vi "计算5针真维度.vi"(2 "引用句柄输入":T2, 3 "Fitted Circle (中间圆)":T1, 4 "Fitted Circle (右下角圆)":T1, 5 "Fitted Circle (左下角圆)":T1, 6 "Fitted Circle (右上角圆)":T1, 7 "Fitted Circle (左上角圆)":T1) -> (1 "Distances":sgl[][](array[numeric]))   [LabVIEW 2014]
uses:
  <vilib>/vision/Image Controls.llb/IMAQ Image.ctl
  <vilib>/vision/NI_Vision_Development_Module.lvlib
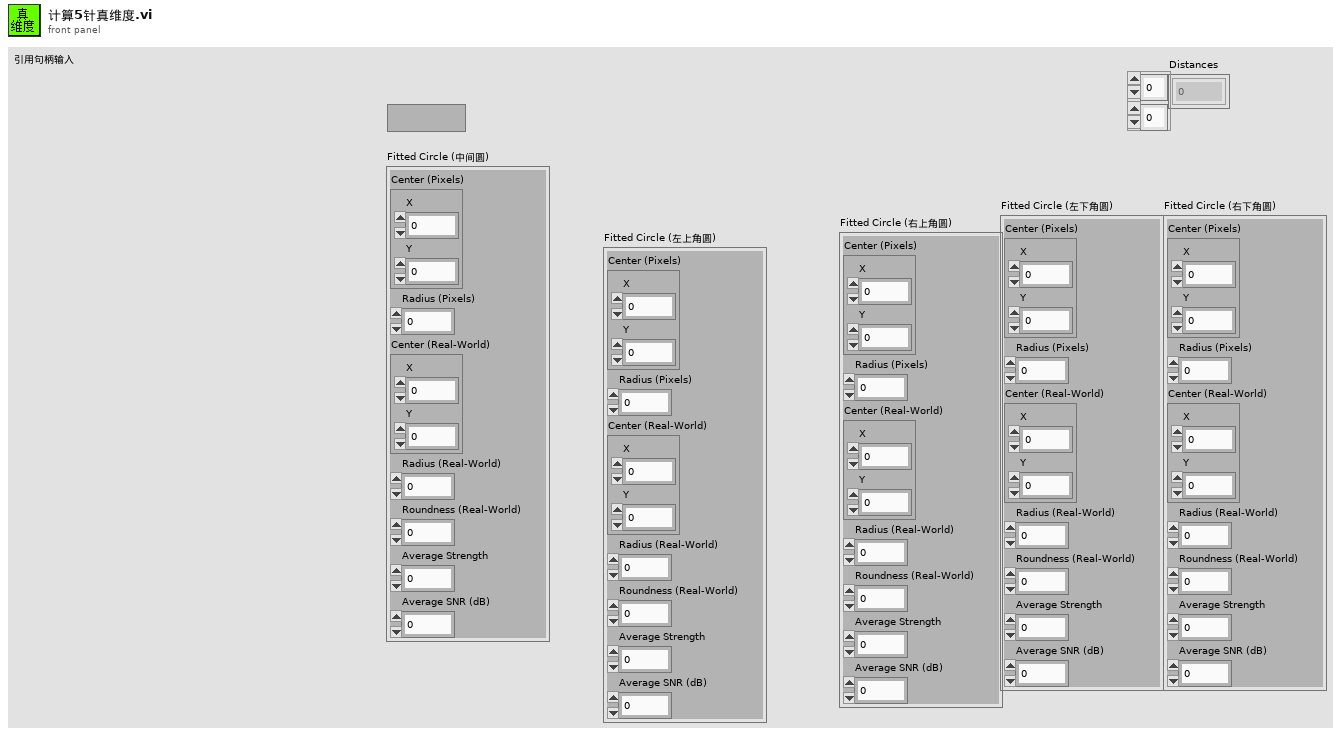
[diagram p1: front panel]
types:
  T1 = cluster{"Center (Pixels)":cluster{"X":sgl, "Y":sgl}, "Radius (Pixels)":dbl, "Center (Real-World)":cluster{"X":sgl, "Y":sgl}, "Radius (Real-World)":dbl, "Roundness (Real-World)":dbl, "Average Strength":dbl, "Average SNR (dB)":dbl}
  T2 = typedef "IMAQ Image.ctl" = refnum<image>
  T3 = cluster{"Center (Pixels)":cluster{"X":sgl, "Y":sgl}, "Radius (Pixels)":dbl, "Center (Real-World)":cluster{"X":sgl, "Y":sgl}, "Radius (Real-World)":dbl, "Roundness (Real-World)":dbl, "Average Strength":dbl, "Average SNR (dB)":dbl}[]
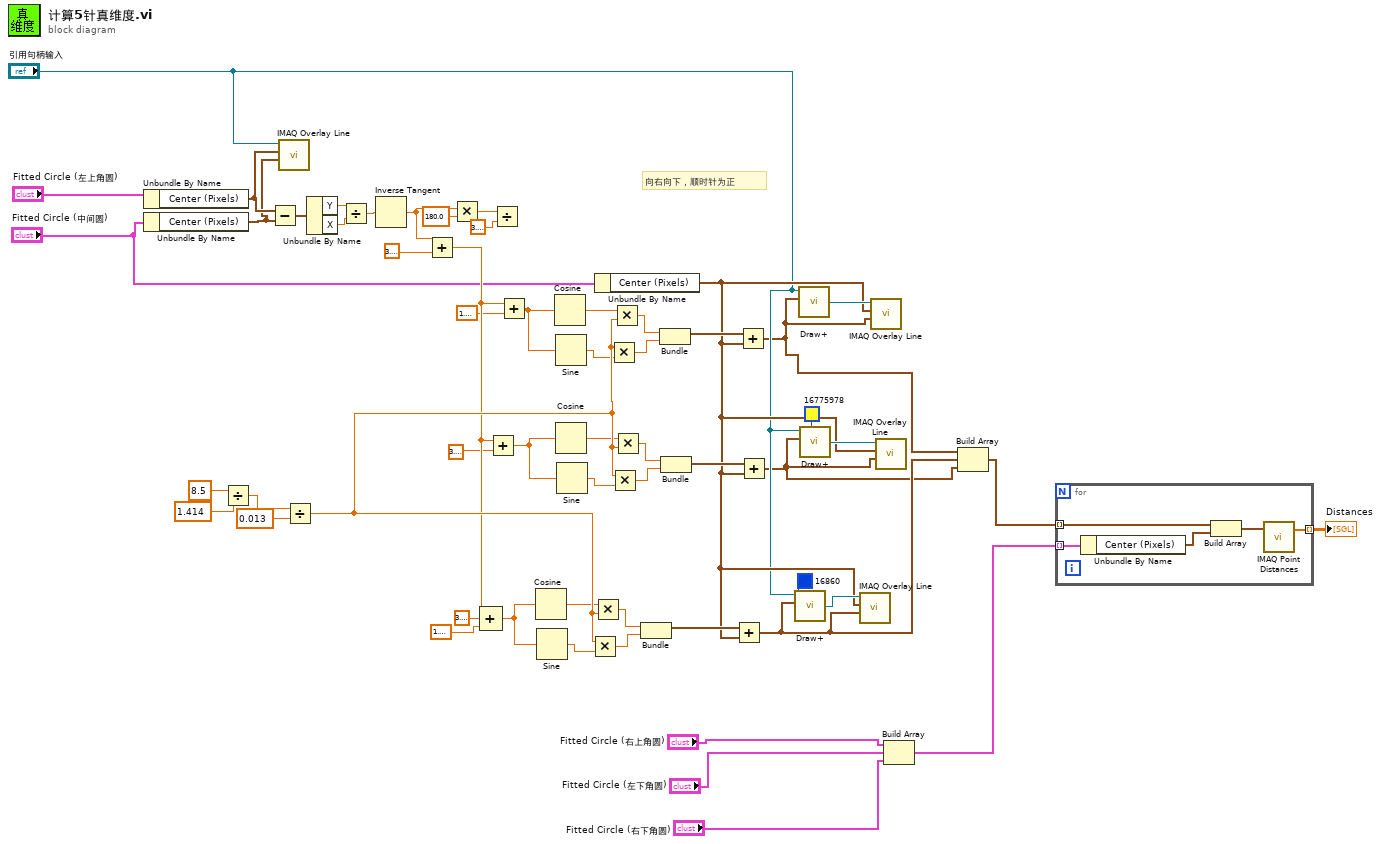
[diagram p0: block diagram]
diagram:
  # "向右向下，顺时针为正"
  n1 = Unbundle By Name("Fitted Circle (左上角圆)") -> ("Center (Pixels)"=w11:cluster{"X":sgl, "Y":sgl})
  n2 = Unbundle By Name("Fitted Circle (中间圆)") -> ("Center (Pixels)"=w10:cluster{"X":sgl, "Y":sgl})
  n3 = Divide(x=8.5, y=1.414) -> (x/y=w26:dbl)
  n4 = Subtract(x=w11, y=w10) -> (x-y=w41:cluster{"X":sgl, "Y":sgl})
  n5 = call "IMAQ Overlay Line"("End Point"=w10, "Start Point"=w11, "Image"="引用句柄输入") -> ()  [unwired: 7 in, 2 out]
  n6 = Divide(x=w26, y=0.013) -> (x/y=w53:dbl)
  n7 = Unbundle By Name(w41) -> ("Y"=w42:sgl, "X"=w43:sgl)
  n8 = Divide(x=w42, y=w43) -> (x/y=w56:sgl)
  n9 = Inverse Tangent(1:w56) -> (0:w57:sgl)
  n10 = Add(x=w57, y=3.141592653589793) -> (x+y=w49:dbl)
  n11 = Multiply(x=w57, y=sgl 180.0) -> (x*y=w19:sgl)
  n12 = Compound Arithmetic op=ADD(w49, 3.141592653589793, 1.5707963267948966) -> (w35:dbl)
  n13 = Add(x=w49, y=3.141592653589793) -> (x+y=w50:dbl)
  n14 = Divide(x=w19, y=3.141592653589793) -> ()  [unwired: 1 out]
  n15 = Add(x=w49, y=1.5707963267948966) -> (x+y=w34:dbl)
  n16 = Cosine(x=w35) -> (cos(x)=w46:dbl)
  n17 = Sine(x=w35) -> (sin(x)=w47:dbl)
  n18 = Cosine(x=w34) -> (cos(x)=w44:dbl)
  n19 = Sine(x=w34) -> (sin(x)=w45:dbl)
  n20 = Cosine(x=w50) -> (cos(x)=w51:dbl)
  n21 = Sine(x=w50) -> (sin(x)=w52:dbl)
  n22 = Multiply(x=w53, y=w47) -> (x*y=w32:dbl)
  n23 = Multiply(x=w46, y=w53) -> (x*y=w31:dbl)
  n24 = Unbundle By Name("Fitted Circle (中间圆)") -> ("Center (Pixels)"=w13:cluster{"X":sgl, "Y":sgl})
  n25 = Multiply(x=w53, y=w45) -> (x*y=w25:dbl)
  n26 = Multiply(x=w53, y=w52) -> (x*y=w54:dbl)
  n27 = Multiply(x=w44, y=w53) -> (x*y=w24:dbl)
  n28 = Multiply(x=w51, y=w53) -> (x*y=w55:dbl)
  n29 = Bundle(w31, w32) -> (w33:cluster{dbl, dbl})  [unwired: 1 in]
  n30 = Bundle(w24, w25) -> (w29:cluster{dbl, dbl})  [unwired: 1 in]
  n31 = Bundle(w55, w54) -> (w30:cluster{dbl, dbl})  [unwired: 1 in]
  n32 = Add(x=w33, y=w13) -> (x+y=w5:cluster{dbl, dbl})
  n33 = Add(x=w29, y=w13) -> (x+y=w6:cluster{dbl, dbl})
  n34 = Add(x=w30, y=w13) -> (x+y=w4:cluster{dbl, dbl})
  n35 = call "Draw+.vi"("Color"=u32 16860, "input cluster"=w5, "Image In"="引用句柄输入") -> ("Image Out"=w15:T2)  [unwired: 3 in]
  n36 = call "Draw+.vi"("input cluster"=w6, "Image In"="引用句柄输入") -> ("Image Out"=w14:T2)  [unwired: 4 in]
  n37 = call "Draw+.vi"("Color"=u32 16775978, "input cluster"=w4, "Image In"="引用句柄输入") -> ("Image Out"=w16:T2)  [unwired: 3 in]
  n38 = call "IMAQ Overlay Line"("End Point"=w5, "Start Point"=w13, "Image"=w15) -> ()  [unwired: 7 in, 2 out]
  n39 = call "IMAQ Overlay Line"("End Point"=w6, "Start Point"=w13, "Image"=w14) -> ()  [unwired: 7 in, 2 out]
  n40 = call "IMAQ Overlay Line"("End Point"=w4, "Start Point"=w13, "Image"=w16) -> ()  [unwired: 7 in, 2 out]
  n41 = Build Array("Fitted Circle (右上角圆)", "Fitted Circle (左下角圆)", "Fitted Circle (右下角圆)") -> (w2:T3)
  n42 = Build Array(w6, w5, w4) -> (w3:cluster{dbl, dbl}[])
  n43 = for {
    tunnel: w3 -> [w62] mode=indexing
    tunnel: w2 -> [w59] mode=indexing
    tunnel: [w58] -> w1 mode=indexing
    n44 = Unbundle By Name(w59) -> ("Center (Pixels)"=w61:cluster{"X":sgl, "Y":sgl})
    n45 = Build Array(w62, w61) -> (w60:cluster{"X":dbl, "Y":dbl}[])
    n46 = call "IMAQ Point Distances"("Points"=w60) -> ("Distances"=w58:sgl[])  [unwired: 4 in, 1 out]
  }
  "Distances" <- w1
